vi "ASI Set ROI Format.vi"(6 "Img_type":i32, 7 "iBin":i32, 9 "iHeight":i32, 10 "iWidth":i32, 11 "iCameraID":i32) -> (3 "function return":i32)   [LabVIEW 2012, in "ASICamera2_no_err.lvlib"]
doc: "ASICAMERA_API ASI_ERROR_CODE ASISetROIFormat(int iCameraID, int iWidth, int iHeight, int iBin, ASI_IMG_TYPE Img_type);"
uses:
  <userlib>/ASICamera2_no_err/ASICamera2_no_err.lvlib
  ASICamera2.dll
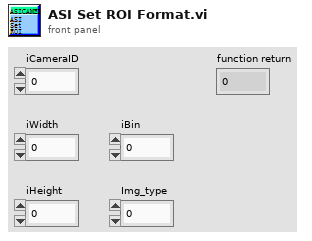
[diagram p1: front panel]
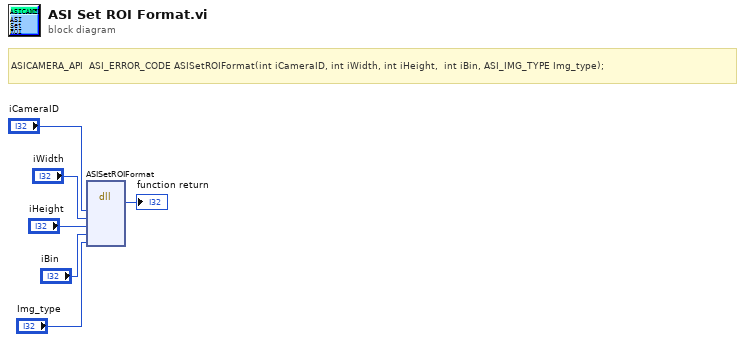
[diagram p0: block diagram]
diagram:
  # "ASICAMERA_API  ASI_ERROR_CODE ASISetROIFormat(int iCameraID, int iWidth, int iHeight,  int iBin, ASI_IMG_TYPE Img_type);"
  n1 = dll-call lib="ASICamera2.*" fn="ASISetROIFormat"("iCameraID"="iCameraID", "iWidth"="iWidth", "iHeight"="iHeight", "iBin"="iBin", "Img_type"="Img_type") -> (→"function return":i32)  [unwired: 8 in, 2 out]
